vi "pack_cluster.vi"(3 "error in":errorcluster, 4 "cluster":variant, 5 "p":u64) -> (0 "error out":errorcluster, 2 "p out":u64)   [LabVIEW 2019, in "msgpack.lvlib"]
doc: "Packs a LabVIEW cluster into the msgpack buffer as a \"map\" object. The keys are the name strings of the cluster, and values the associated cluster values."
uses:
  msgpack.lvlib
panel:
  # "msgpack"
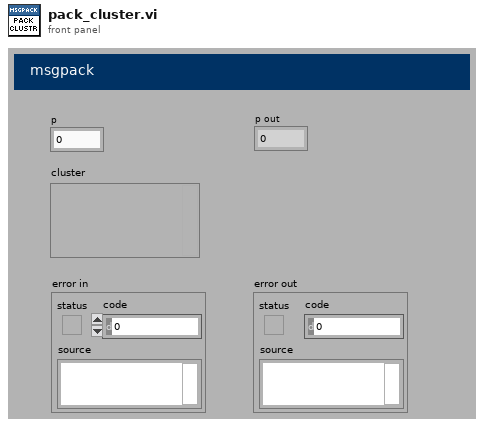
[diagram p1: front panel]
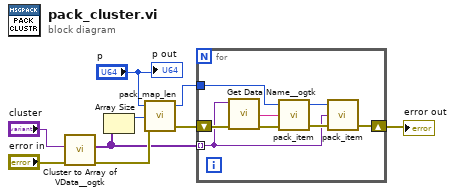
[diagram p0: block diagram]
diagram:
  n1 = call "Cluster to Array of VData__ogtk.vi"("error in (no error)"="error in", "Cluster"="cluster") -> ("error out"=w9:errorcluster, "Array of VData"=w7:variant[])  [unwired: 8 in]
  n2 = Array Size(array=w7) -> (size(s)=w6:i32)
  n3 = call "pack_map_len.vi"("error in"=w9, "n"=w6, "p"="p") -> ("error out"=w8:errorcluster, "p out"=w5:u64)  [unwired: 1 in]
  n4 = for {
    shift-right: [w13] -> w2
    shift-left: w8 -> [w17]
    tunnel: w7 -> [w12] mode=indexing
    tunnel: w5 -> [w11]
    n5 = call "Get Data Name__ogtk.vi"("error in (no error)"=w17, "Data"=w12) -> ("error out"=w16:errorcluster, "Data Name"=w15:string)  [unwired: 7 in, 1 out]
    n6 = call "pack_item.vi"("error in"=w16, "x"=w15, "p"=w11) -> ("error out"=w14:errorcluster, "p out"=w10:u64)  [unwired: 1 in]
    n7 = call "pack_item.vi"("error in"=w14, "x"=w12, "p"=w10) -> ("error out"=w13:errorcluster)  [unwired: 1 in, 1 out]
  }
  "error out" <- w2
  "p out" <- "p"
